vi "Set Default.vi"(8 "error in (no error)":errorcluster, 11 "List Driver Aliases Msg in":refnum<class "List Driver Aliases Msg.lvclass">) -> (0 "error out":errorcluster, 3 "List Driver Aliases Msg out":refnum<class "List Driver Aliases Msg.lvclass">)   [LabVIEW 2020, in "Instrument Handler.lvlib" / "List Driver Aliases Msg.lvclass"]
doc: "Restore private data to a defined default state.\n\nThis implementation sets:\nPublish = FALSE\nAwait reply with -1 in timeout"
uses:
  List Driver Aliases Msg.lvclass
  C:/Current projects/WS/Framework/Framework/Actors/Instrument Handler/Instrument Handler Messages/Instrument Handler Response Msg/Instrument Handler Response Msg.lvclass
  PPL/HDH.Actor Framework.Core.Publisher.lvlibp/Messages/Response Msg/Response Core/Controls/Ctl_SendFunction.ctl
  Instrument Handler Response Msg/Instrument Handler Response Msg.lvclass/Instrument Handler Response Msg.ctl
  Instrument Handler Response Msg/Instrument Handler Response Msg.lvclass
  PPL/HDH.Actor Framework.Core.Publisher.lvlibp
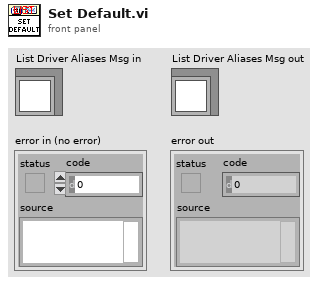
[diagram p1: front panel]
types:
  T1 = typedef "HDH.Actor Framework.Core.Publisher.lvlibp/Ctl_SendFunction.ctl" = enum16{"Send and Forget", "Request Reply", "Await Reply"}
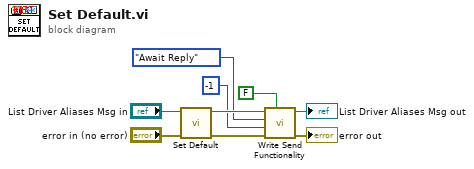
[diagram p0: block diagram]
diagram:
  n1 = call-parent "Set Default.vi"("error in (no error)"="error in (no error)", "Flex Msg in"="List Driver Aliases Msg in") -> ("error out"=w5:errorcluster, "Flex Msg out"=w7:refnum<class "List Driver Aliases Msg.lvclass">)  [unwired: 8 in]
  n2 = call "Write Send Functionality.vi"("Publish Data?(T)"=FALSE, "error in (no error)"=w5, "Timeout if Waiting(-1ms)"=-1, "Send Function(Await Reply)"=Ctl_SendFunction."Await Reply", "Instrument Handler Reponse Msg in"=w7) -> ("error out"=→"error out":errorcluster, "Instrument Handler Reponse Msg out"=→"List Driver Aliases Msg out":refnum<class "List Driver Aliases Msg.lvclass">)  [unwired: 5 in]
